vi "Generate Thermal Test Cases.vi"() -> (2 "Array":refnum<class "Thermal Test.lvclass">[](array[class]))   [LabVIEW 2023]
uses:
  Thermal Test/Thermal Test.lvclass
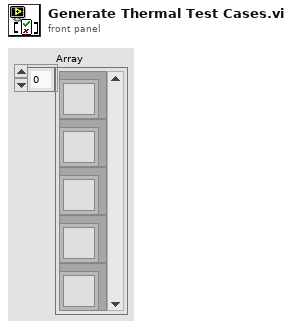
[diagram p1: front panel]
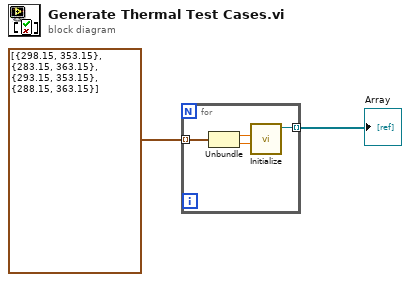
[diagram p0: block diagram]
diagram:
  n1 = for {
    tunnel: cluster{dbl[unit], dbl[unit]}[] [{298.15, 353.15}, {283.15, 363.15}, {293.15, 353.15}, {288.15, 363.15}] -> [w6] mode=indexing
    tunnel: [w3] -> w1 mode=indexing
    n2 = Unbundle(w6) -> (w5:dbl[unit], w4:dbl[unit])
    n3 = call "Initialize.vi"("max ending temperature"=w4, "starting temperature"=w5) -> ("Thermal Test out"=w3:refnum<class "Thermal Test.lvclass">)  [unwired: 9 in]
  }
  "Array" <- w1
